vi "GetWhileLoopReference.vi"(8 "error in":errorcluster, 11 "WhileLoop in":refnum<class "WhileLoop.lvclass">) -> (0 "error out":errorcluster, 1 "reference out":refnum<vi>, 3 "WhileLoop out":refnum<class "WhileLoop.lvclass">)   [LabVIEW 2014, in "Raspberry Pi Compatible Compiler for LabVIEW.lvlib" / "WhileLoop.lvclass"]
uses:
  WhileLoop.lvclass
  Generic/Generic.lvclass
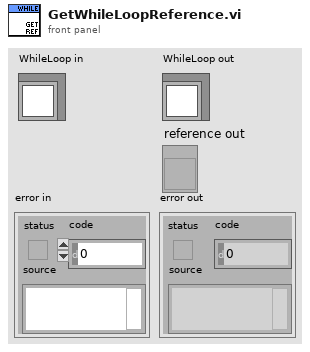
[diagram p1: front panel]
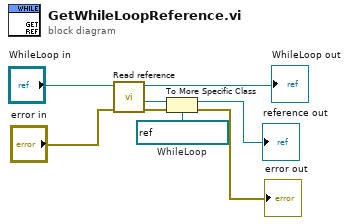
[diagram p0: block diagram]
diagram:
  w6 = refnum<vi> refnum  # WhileLoop
  n1 = call "Read reference.vi"("error in"="error in", "GObject in"="WhileLoop in") -> ("error out"=w7:errorcluster, "reference"=w8:refnum<vi>, "GObject out"=→"WhileLoop out":refnum<class "WhileLoop.lvclass">)  [unwired: 5 in]
  n2 = To More Specific Class(target class=w6, reference=w8, error in=w7) -> (specific class reference=→"reference out":refnum<vi>, error out=→"error out":errorcluster)
